vi "CVT2GroupNotFoundTest.vi"() -> (3 "Unit Test Framework Results":T1)   [LabVIEW 2013, in "UnitTests.lvlib"]
uses:
  UnitTests.lvlib
  <vilib>/utf/common/utf_test_result_troll.ctl
  <vilib>/utf/common/utf_test_result.ctl
  <vilib>/utf/common/utf_test_result_failure.ctl
  <vilib>/utf/common/utf_test_comparison_operators.ctl
  <vilib>/utf/common/utf_vi_tag.ctl
  <vilib>/NI/Current Value Table/Read tags into grouped data.vi
  <vilib>/NI/Current Value Table/Read Index Set.vi
  <vilib>/NI/Current Value Table/DataTypes/Double_Read Index Set.vi
  <vilib>/NI/Current Value Table/DataTypes/Array of String_Read Index Set.vi
  <vilib>/NI/Current Value Table/DataTypes/Array of Boolean_Read Index Set.vi
  <vilib>/NI/Current Value Table/DataTypes/Array of Single_Read Index Set.vi
  <vilib>/NI/Current Value Table/DataTypes/Array of Double_Read Index Set.vi
  <vilib>/NI/Current Value Table/DataTypes/Array of I8_Read Index Set.vi
  <vilib>/NI/Current Value Table/DataTypes/Array of I16_Read Index Set.vi
  <vilib>/NI/Current Value Table/DataTypes/Array of I32_Read Index Set.vi
  <vilib>/NI/Current Value Table/DataTypes/Array of I64_Read Index Set.vi
  <vilib>/NI/Current Value Table/DataTypes/Array of U64_Read Index Set.vi
  <vilib>/NI/Current Value Table/DataTypes/Array of U32_Read Index Set.vi
  <vilib>/NI/Current Value Table/DataTypes/Array of U16_Read Index Set.vi
  <vilib>/NI/Current Value Table/DataTypes/Array of U8_Read Index Set.vi
  <vilib>/NI/Current Value Table/DataTypes/Boolean_Read Index Set.vi
  <vilib>/NI/Current Value Table/DataTypes/String_Read Index Set.vi
  <vilib>/NI/Current Value Table/DataTypes/U8_Read Index Set.vi
  <vilib>/NI/Current Value Table/DataTypes/U16_Read Index Set.vi
  <vilib>/NI/Current Value Table/DataTypes/U32_Read Index Set.vi
  <vilib>/NI/Current Value Table/DataTypes/U64_Read Index Set.vi
  <vilib>/NI/Current Value Table/DataTypes/I8_Read Index Set.vi
  <vilib>/NI/Current Value Table/DataTypes/I16_Read Index Set.vi
  <vilib>/NI/Current Value Table/DataTypes/I32_Read Index Set.vi
  <vilib>/NI/Current Value Table/DataTypes/I64_Read Index Set.vi
  <vilib>/NI/Current Value Table/DataTypes/Single_Read Index Set.vi
  <vilib>/NI/Current Value Table/FGVs/Group Memory.vi
  <vilib>/NI/Current Value Table/Memory Block.vi
  <vilib>/NI/Current Value Table/DataTypes/Double_Memory Block.vi
  <vilib>/NI/Current Value Table/DataTypes/Array of String_Memory Block.vi
  <vilib>/NI/Current Value Table/DataTypes/Array of Boolean_Memory Block.vi
  <vilib>/NI/Current Value Table/DataTypes/Array of Single_Memory Block.vi
  <vilib>/NI/Current Value Table/DataTypes/Array of Double_Memory Block.vi
  <vilib>/NI/Current Value Table/DataTypes/Array of I8_Memory Block.vi
  <vilib>/NI/Current Value Table/DataTypes/Array of I16_Memory Block.vi
  <vilib>/NI/Current Value Table/DataTypes/Array of I32_Memory Block.vi
  <vilib>/NI/Current Value Table/DataTypes/Array of I64_Memory Block.vi
  <vilib>/NI/Current Value Table/DataTypes/Array of U64_Memory Block.vi
  <vilib>/NI/Current Value Table/DataTypes/Array of U32_Memory Block.vi
  <vilib>/NI/Current Value Table/DataTypes/Array of U16_Memory Block.vi
  <vilib>/NI/Current Value Table/DataTypes/Array of U8_Memory Block.vi
  <vilib>/NI/Current Value Table/DataTypes/Boolean_Memory Block.vi
  <vilib>/NI/Current Value Table/DataTypes/String_Memory Block.vi
  <vilib>/NI/Current Value Table/DataTypes/U8_Memory Block.vi
  <vilib>/NI/Current Value Table/DataTypes/U16_Memory Block.vi
  <vilib>/NI/Current Value Table/DataTypes/U32_Memory Block.vi
  <vilib>/NI/Current Value Table/DataTypes/U64_Memory Block.vi
  <vilib>/NI/Current Value Table/DataTypes/I8_Memory Block.vi
  <vilib>/NI/Current Value Table/DataTypes/I16_Memory Block.vi
  <vilib>/NI/Current Value Table/DataTypes/I32_Memory Block.vi
  <vilib>/NI/Current Value Table/DataTypes/I64_Memory Block.vi
  <vilib>/NI/Current Value Table/DataTypes/Single_Memory Block.vi
  <vilib>/utf/NI_UnitTestFramework.lvlib
  <vilib>/NI/Current Value Table/Current Value Table.lvlib
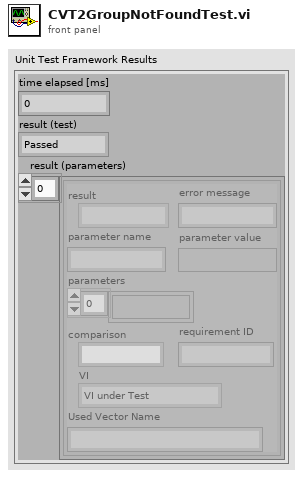
[diagram p1: front panel]
types:
  T1 = typedef "NI_UnitTestFramework.lvlib/utf_test_result_troll.ctl" = cluster{"time elapsed [ms]":u32, "result (test)":T2, "result (parameters)":T3[]}
  T2 = typedef "NI_UnitTestFramework.lvlib/utf_test_result.ctl" = enum16{"Passed", "Failed", "Error", "Skipped", "Not Processed"}
  T3 = typedef "NI_UnitTestFramework.lvlib/utf_test_result_failure.ctl" = cluster{"result":T2, "error message":string, "parameter name":string, "parameter value":variant, "parameters":variant[], "comparison":T4, "requirement ID":string, "VI":T5, "Used Vector Name":string}
  T4 = typedef "NI_UnitTestFramework.lvlib/utf_test_comparison_operators.ctl" = enum16{"=", "!=", ">", ">=", "<", "<=", "range", "symmetric tolerance", "asymmetric tolerance", "string contains", "string not contain", "array size", "string length", "array range", "by element", "array range (limit array)", "user-defined", "array contains", "array not contain", "vector length", "= (elm)", "!= (elm)", "= (case insensitive)", "!= (case insensitive)"}
  T5 = typedef "NI_UnitTestFramework.lvlib/utf_vi_tag.ctl" = enum16{"Setup VI", "VI under Test", "Teardown VI"}
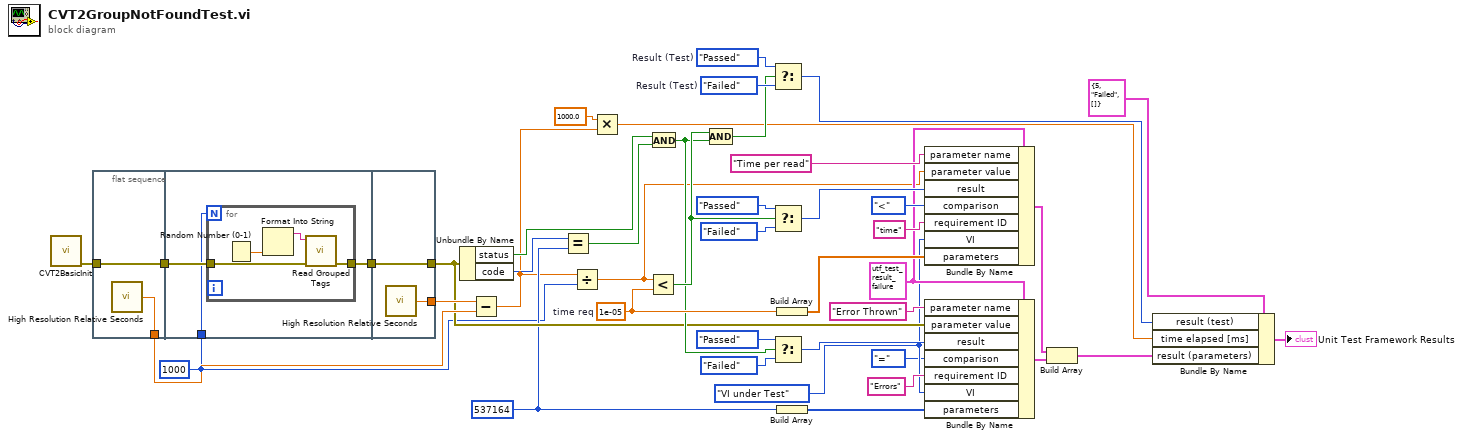
[diagram p0: block diagram]
diagram:
  w2 = 1000
  w15 = utf_test_result."Passed"  # Result (Test)
  w16 = utf_test_result."Failed"  # Result (Test)
  w7 = 537164 ("y")
  w5 = utf_vi_tag."VI under Test" ("VI")
  w29 = 1e-05  # time req
  w27 = T3 {"result"=enum."Passed", "error message"="", "parameter name"="", "parameter value"=variant, "parameters"=[], "comparison"=enum."=", "requirement ID"="", "VI"=enum."Setup VI", "Used Vector Name"=""} ("Unit Test Framework - result (parameters)")
  n1 = call "CVT2BasicInit.vi"() -> ("error out"=w39:errorcluster)  [unwired: 9 in, 2 out]
  n2 = flat-sequence {
    tunnel: [w45] -> w40
    tunnel: w39 -> [w44]
    tunnel: [w44] -> w38
    tunnel: w38 -> [w48]
    tunnel: [w47] -> w37
    tunnel: w2 -> [w46]
    tunnel: [w54] -> w41
    tunnel: [w53] -> w9
    tunnel: w37 -> [w53]
    frame #0 {
      n3 = call <vilib>:"High Resolution Relative Seconds.vi"() -> ("relative seconds"=w45:dbl)
    }
    frame #1 {
      n4 = for {
        N: w46 -> [_]
        tunnel: w48 -> [w50]
        tunnel: [w51] -> w47
        n5 = Random Number (0-1)() -> (number: 0 to 1=w52:dbl)
        n6 = Format Into String(w52) -> (resulting string=w49:string)  [unwired: 3 in, 1 out]
        n7 = call <vilib>:"Read Grouped Tags.vi"("error in (no error)"=w50, "Group"=w49) -> ("error out"=w51:errorcluster)  [unwired: 8 in, 1 out]
      }
    }
    frame #2 {
      n8 = call <vilib>:"High Resolution Relative Seconds.vi"() -> ("relative seconds"=w54:dbl)
    }
  }
  n9 = Unbundle By Name(w9) -> ("status"=w21:bool, "code"=w23:i32)
  n10 = Subtract(x=w41, y=w40) -> (x-y=w3:dbl)
  n11 = Equal?(x=w23, y=w7) -> (x = y?=w22:bool)
  n12 = Divide(x=w3, y=w2) -> (x/y=w1:dbl)
  n13 = Multiply(x=1000.0 ("y"), y=w3) -> (x*y=w12:dbl)
  n14 = Less?(x=w1, y=w29) -> (x < y?=w18:bool)
  n15 = And(x=w21, y=w22) -> (x .and. y?=w17:bool)
  n16 = Compound Arithmetic op=AND(w18, w17) -> (w14:bool)
  n17 = Select(t=w15, s=w14, f=w16) -> (s? t:f=w13:T2)
  n18 = Select(t=utf_test_result."Passed" ("result"), s=w18, f=utf_test_result."Failed" ("result")) -> (s? t:f=w31:T2)
  n19 = Select(t=utf_test_result."Passed" ("result"), s=w17, f=utf_test_result."Failed" ("result")) -> (s? t:f=w10:T2)
  n20 = Build Array(w29) -> (w30:dbl[])
  n21 = Build Array(w7) -> (w8:i32[])
  n22 = Bundle By Name(cluster=w27, "parameter name"="Time per read", "parameter value"=w1, "result"=w31, "comparison"=utf_test_comparison_operators."<", "requirement ID"="time", "VI"=w5, "parameters"=w30) -> (w26:T3)
  n23 = Bundle By Name(cluster=w27, "parameter name"="Error Thrown", "parameter value"=w9, "result"=w10, "comparison"=utf_test_comparison_operators."=", "requirement ID"="Errors" ("parameter name"), "VI"=w5, "parameters"=w8) -> (w25:T3)
  n24 = Build Array(w26, w25) -> (w11:T3[])
  n25 = Bundle By Name(cluster=T1 {"time elapsed [ms]"=5, "result (test)"=enum."Failed", "result (parameters)"=[]} ("Unit Test Framework - Result"), "result (test)"=w13, "time elapsed [ms]"=w12, "result (parameters)"=w11) -> (→"Unit Test Framework Results":T1)
